vi "winston-authentication-example.vi"() -> ()   [LabVIEW 2017]
uses:
  <vilib>/httpClient/POSTBuffer.vi
  <vilib>/httpClient/LabVIEWHTTPClient.lvlib
panel:
  out "error out":errorcluster
  out "jwtToken":string="eyJhbGciOiJIUzI1NiIsInR5cCI6IkpXVCJ9.eyJkYXRhIjp7ImNsaWVudFNlcmlhbCI6ImRldmVsb3BlciIsImxpY2Vuc2VWYWxpZFVudGlsIjoiMTg5NzkxODUyNjAwMCJ9LCJpYXQiOjE1ODIzMDAyMjksImV4cCI6MTU4MjM4NjYyOX0.iY-YLVVzkOAtTILYIx_1T5l_p0eZNRgwxAISscrqsL8"
  in  "clientSerial":string="developer"
  in  "licenseHash":string
  in  "url":string="https://gikr1vhulg.execute-api.eu-west-1.amazonaws.com/playground/v1/auth/client"
  in  "API key":string
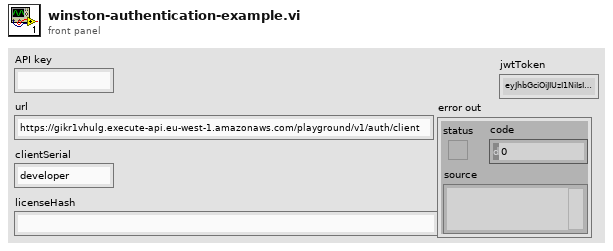
[diagram p1: front panel]
types:
  T1 = cluster{"clientSerial":string, "licenseHash":string}
  T2 = typedef "LabVIEWHTTPClient.lvlib/ClientHandle.ctl" = refnum<k1>
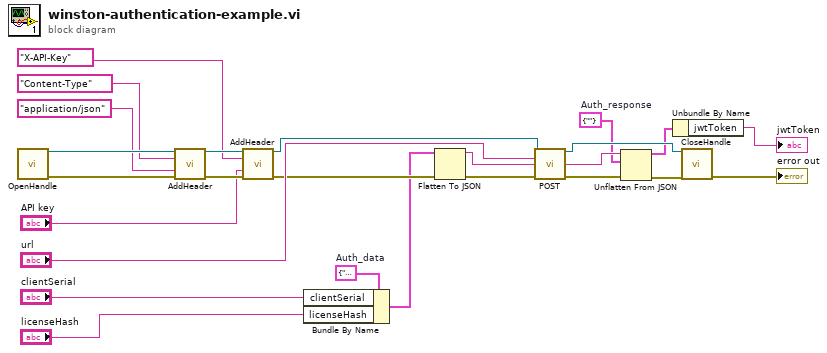
[diagram p0: block diagram]
diagram:
  w12 = cluster{"jwtToken":string} {"jwtToken"=""}  # Auth_response
  w16 = T1 {"clientSerial"="", "licenseHash"=""}  # Auth_data
  n1 = call <vilib>:"OpenHandle.vi"() -> ("client handle out"=w25:T2, "error out"=w24:errorcluster)  [unwired: 14 in]
  n2 = call <vilib>:"AddHeader.vi"("client handle"=w25, "header"="Content-Type", "value"="application/json", "error in (no error)"=w24) -> ("client handle out"=w21:T2, "error out"=w20:errorcluster)  [unwired: 10 in]
  n3 = call <vilib>:"AddHeader.vi"("client handle"=w21, "header"="X-API-Key", "value"="API key", "error in (no error)"=w20) -> ("client handle out"=w7:T2, "error out"=w9:errorcluster)  [unwired: 10 in]
  n4 = Bundle By Name(cluster=w16, "clientSerial"="clientSerial", "licenseHash"="licenseHash") -> (w2:T1)
  n5 = Flatten To JSON(anything=w2, error in (no error)=w9) -> (JSON string=w15:string, 11:w8:errorcluster)  [unwired: 1 in]
  n6 = call-poly <vilib>:"POST.vi"("client handle"=w7, "url"="url", "buffer"=w15, "error in (no error)"=w8) -> ("client handle out"=w14:T2, "body"=w13:string, "error out"=w6:errorcluster)  [unwired: 8 in, 1 out]
  n7 = Unflatten From JSON(JSON string=w13, type and defaults=w12, error in (no error)=w6) -> (value=w11:cluster{"jwtToken":string}, error out=w5:errorcluster)  [unwired: 4 in]
  n8 = Unbundle By Name(w11) -> ("jwtToken"=→"jwtToken":string)
  n9 = call <vilib>:"CloseHandle.vi"("client handle"=w14, "error in (no error)"=w5) -> ("error out"=→"error out":errorcluster)  [unwired: 13 in]
